vi "Main.vi"() -> ()   [LabVIEW 2020]
panel:
  in  "baud rate (9600)":u32=9600
  in  "VISA resource name":refnum<visa-resource-name>
  out "error out":errorcluster
  in  "error in (no error)":errorcluster
  in  "MenosZ":bool
  in  "MenosY":bool
  in  "MenosX":bool
  in  "MenosGarra":bool
  in  "MaisZ":bool
  in  "MaisY":bool
  in  "MaisX":bool
  in  "MaisGarra":bool
  in  "Stop":bool
  out "Status":string
  in  "PIDs":bool
  in  "Configuracao":bool
  in  "Calibracao":bool
  in  "Velocidade [°/s]":dbl[unit](knob) caption="Velocidade" scale=10.0..100.0
  out "Pos10":bool
  out "Pos9":bool
  out "Pos8":bool
  out "Pos7":bool
  out "Pos6":bool
  out "Pos5":bool
  out "Pos4":bool
  out "Pos3":bool
  out "Pos2":bool
  out "Pos1":bool
  in  "GravarAtual":bool
  in  "Start":bool
  in  "ApagarAnterior":bool
  in  "Servo On":bool
  out "ZProgress":u8(slide) scale=0.0..100.0
  out "YProgress":u8(slide) scale=0.0..100.0
  out "XProgress":u8(slide) scale=0.0..100.0
  out "GarraProgress":u8(slide) scale=0.0..100.0
  out "Z":string
  out "Y":string
  out "X":string
  out "Garra":string
  in  "Habilitar controle":enum32{"Item 0", "Item 1"}(radio)
  in  "Modo de Operação":enum32{"Item 0", "Item 1"}(radio)
  # "Projeto Integrador"
  # "Tecnologia em Mecatrônica Industrial - 2020"
  # "Ciclo Automático"
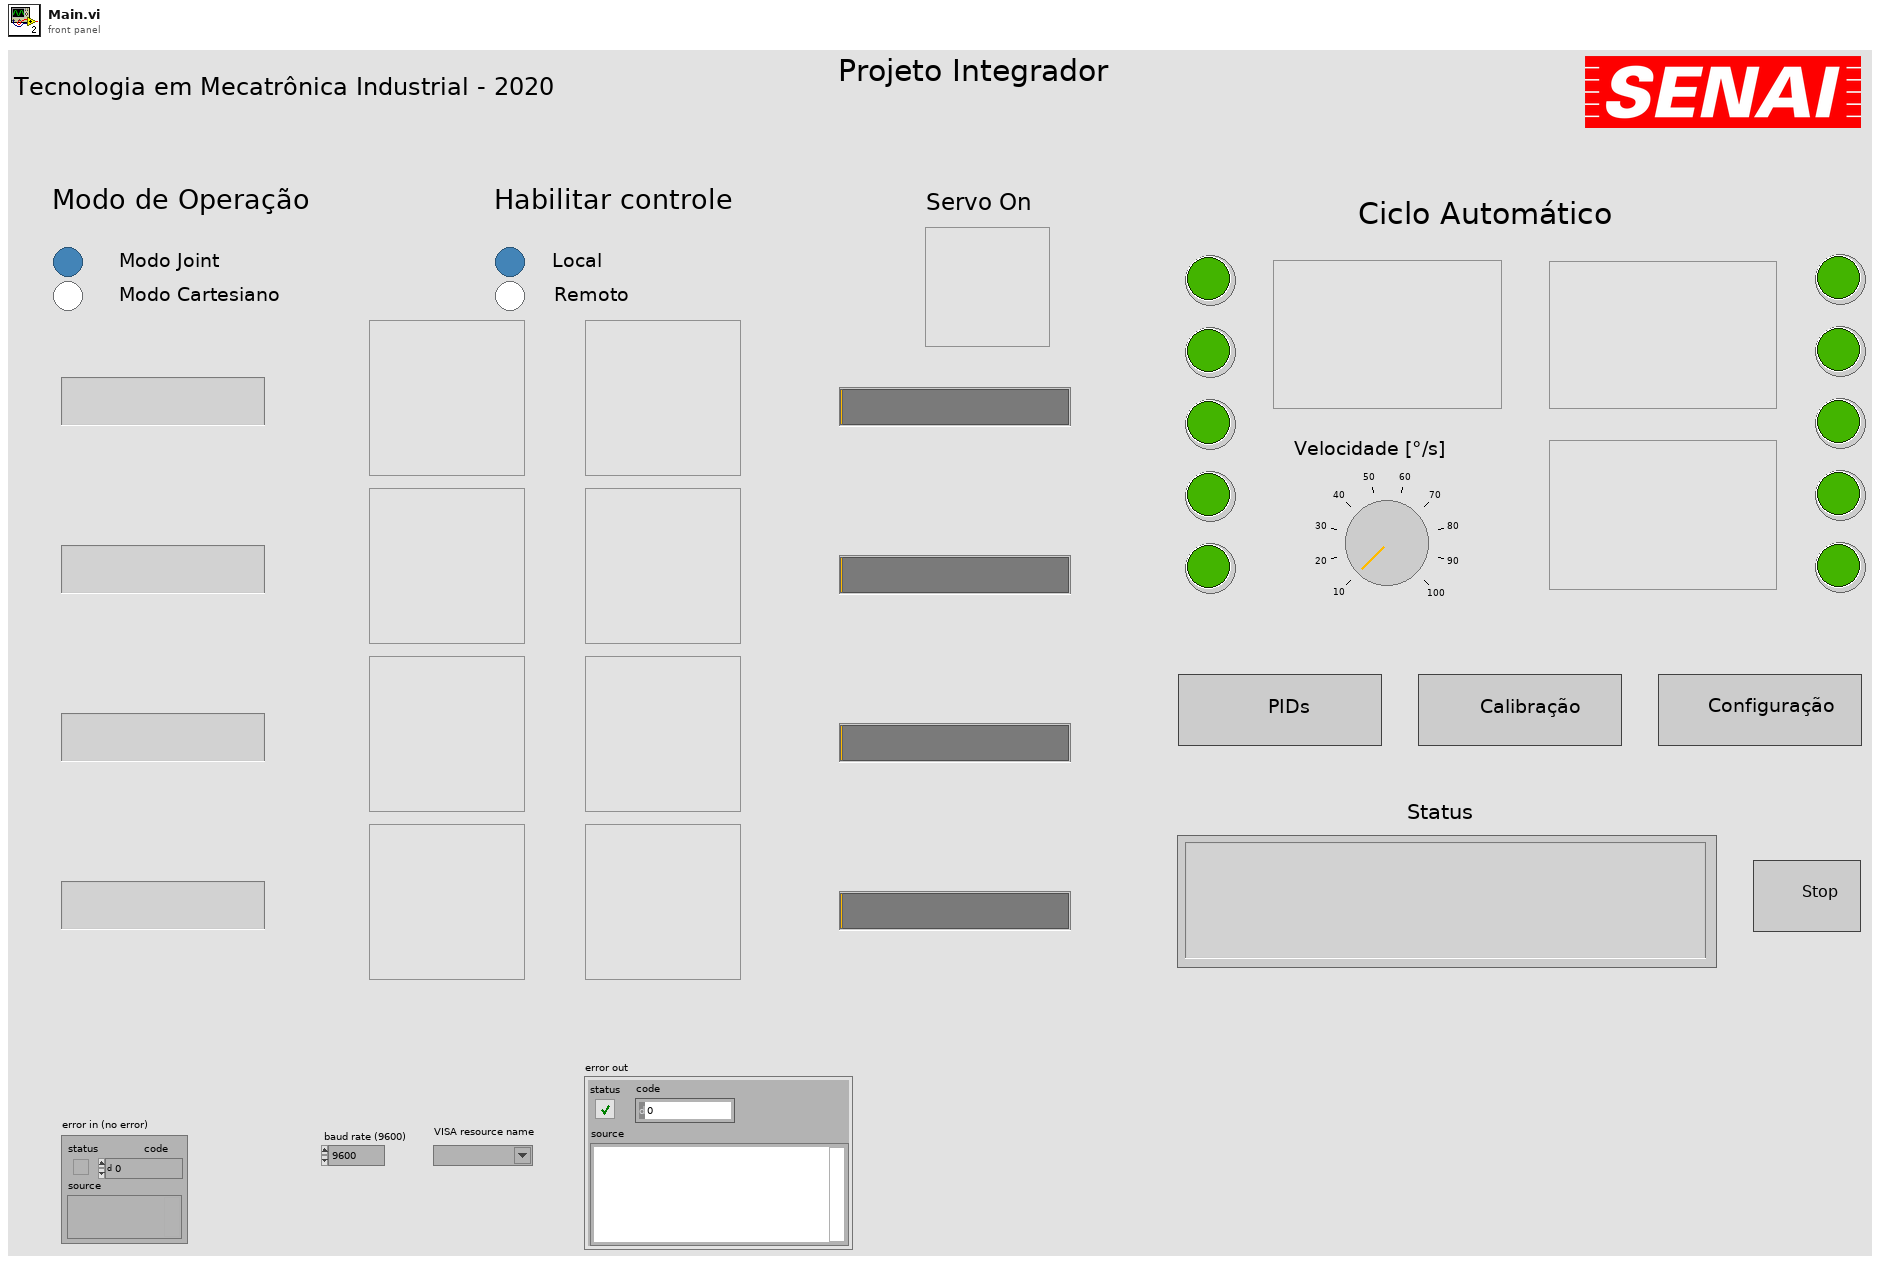
[diagram p1: front panel]
types:
  T1 = enum16{"Init", "G+", "G-", "X+", "X-", "Y+", "Y-", "Z+", "Z-", ""}
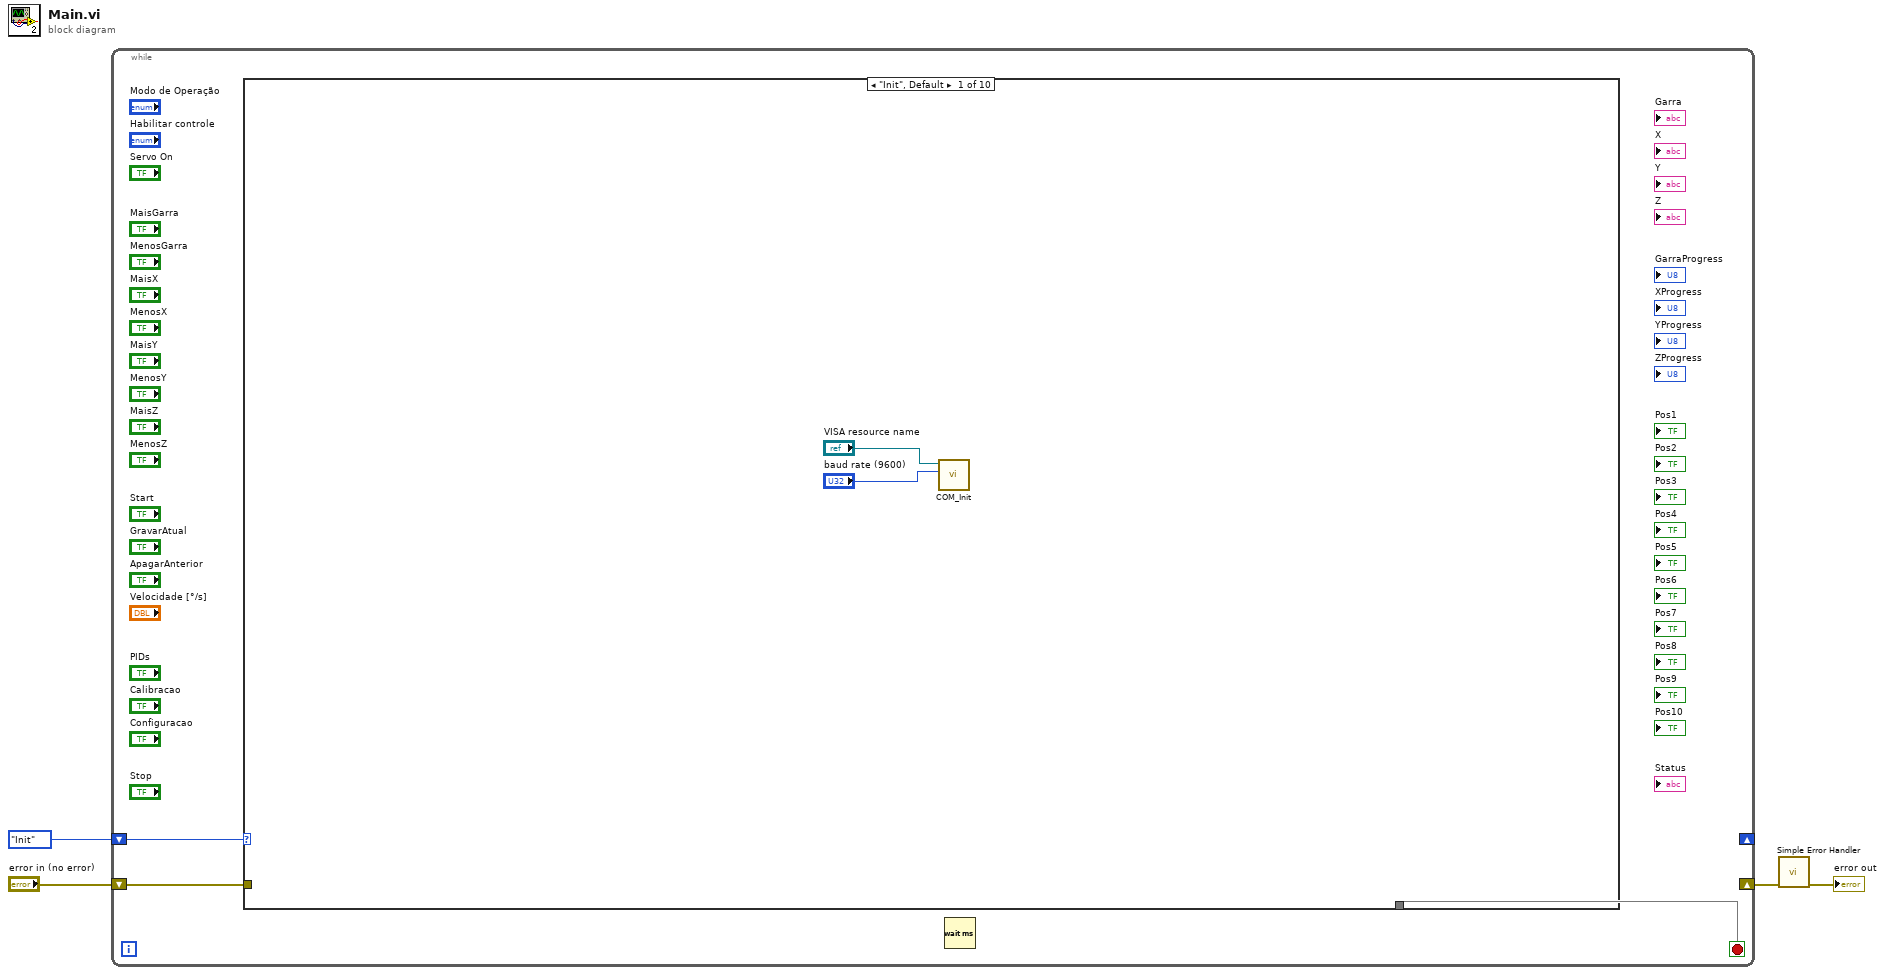
[diagram p0: block diagram]
diagram:
  n1 = while {
    shift-right: _ -> [_]
    shift-left: T1."Init" ("Enum") -> [w7]
    shift-right: [_] -> w1
    shift-left: "error in (no error)" -> [w6]
    stop <- w5 stop-if-true
    n2 = case shown="\"Init\", Default" w7 {
      tunnel: w6 -> [_ _ _ _ _ _ _ _ _ _]
      tunnel: [_ _ _ _ _ _ _ _ _ _] -> w5
      frame "Init", Default {
        n3 = call "COM_Init.vi"("baud rate (9600)"="baud rate (9600)", "VISA Refnum in"="VISA resource name") -> ()  [unwired: 8 in, 2 out]
      }
      frame "G+" {
      }
      frame "G-" {
      }
      frame "X+" {
      }
      frame "X-" {
      }
      frame "Y+" {
      }
      frame "Y-" {
      }
      frame "Z+" {
      }
      frame "Z-" {
      }
      frame "" {
      }
    }
    n4 = Wait (ms)() -> ()  [unwired: 1 in, 1 out]
  }
  n5 = call <vilib>:"Simple Error Handler.vi"("error in (no error)"=w1) -> ("error out"=→"error out":errorcluster)  [unwired: 4 in, 4 out]
